vi "Start Regs.vi"(8 "error in (no error)":errorcluster, 9 "Regs_Descriptions":string[][](array[string]), 10 "RegsParam":dbl[][](array[numeric]), 11 "Queue in":T1) -> (0 "error out":errorcluster)   [LabVIEW 2019, in "Reg visu.lvclass"]
uses:
  Reg visu/Reg visu.lvclass
  <vilib>/NI/AMC/Message Queue.ctl
  <vilib>/NI/AMC/Message.ctl
  <vilib>/NI/Tools/Keyed Array/KeyedArray.ctl
  Reg visu/Reg visu.lvclass/Reg visu.ctl
  Reg visu/Run.vi
  <vilib>/NI/Tools/Keyed Array/Tools_KeyedArray.lvlib
  <vilib>/NI/AMC/AMC.lvlib
panel:
  # "group"
  # "process_gas"
  # "fcode"
  # "fcode_full"
  # "instrument_range_max"
  # "auto_value"
  # "alr_value"
  # "output_k"
  # "output_set_time"
  # "process_units"
  # "Names"
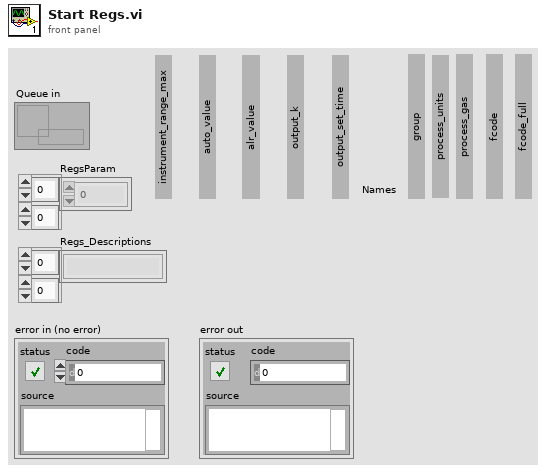
[diagram p1: front panel]
types:
  T1 = typedef "AMC.lvlib/Message Queue.ctl" = refnum<queue>
  T2 = enum32{"Invalid", "Standard", "Closed", "Hidden", "Minimized", "Maximized"}
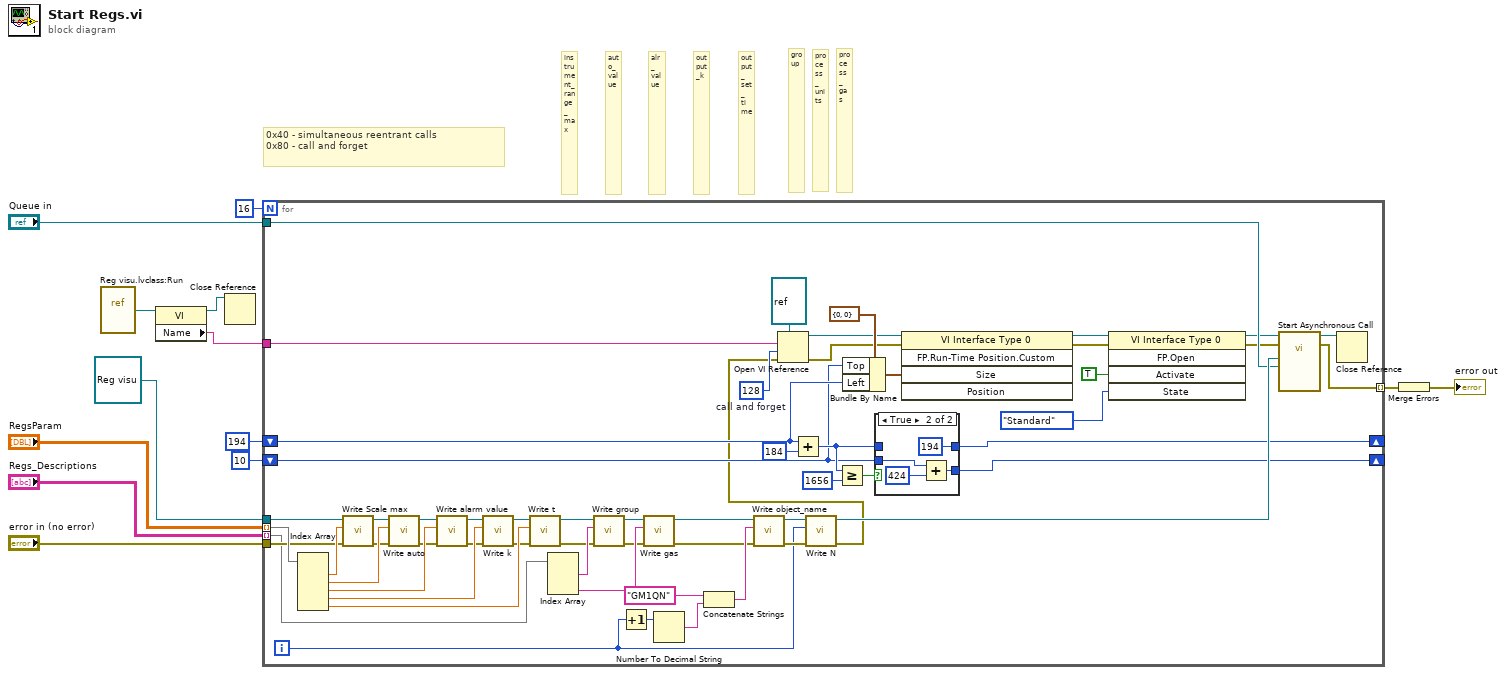
[diagram p0: block diagram]
diagram:
  # "process_gas"
  # "group"
  # "process_units"
  # "output_set_time"
  # "output_k"
  # "alr_value"
  # "instrument_range_max"
  # "auto_value"
  # "0x40 - simultaneous reentrant calls\n0x80 - call and forget"
  n1 = vi-ref "Reg visu.lvclass:Run.vi"() -> (w8:refnum<vi>)
  n2 = property class="VI"(reference=w8) -> (reference out=w7:refnum<vi>, "Name"=w3:string)  [unwired: 1 in, 1 out]
  n3 = Close Reference(reference=w7) -> ()  [unwired: 1 in, 1 out]
  n4 = for {
    N: 16 -> [_]
    tunnel: [w71] -> w9 mode=indexing
    tunnel: refnum<class "Reg visu.lvclass"> refnum ("Reg visu.lvclass") -> [w14]
    tunnel: "Queue in" -> [w63]
    shift-right: [w48] -> _
    shift-left: i16 194 ("x") -> [w50]
    shift-right: [w47] -> _
    shift-left: i16 10 ("x") -> [w49]
    tunnel: "error in (no error)" -> [w32]
    tunnel: w3 -> [w44]
    tunnel: "RegsParam" -> [w34] mode=indexing
    tunnel: "Regs_Descriptions" -> [w23] mode=indexing
    i -> [w64]
    w45 = 128  # call and forget
    n5 = Index Array(array=w34) -> (element #1=w33:dbl, element #2=w31:dbl, element #3=w29:dbl, element #4=w27:dbl, element #5=w25:dbl)  [unwired: 5 in]
    n6 = call "Write Scale max.vi"("error in (no error)"=w32, "Scale max"=w33, "Reg visu in"=w14) -> ("error out"=w30:errorcluster, "Reg visu out"=w38:refnum<class "Reg visu.lvclass">)  [unwired: 7 in]
    n7 = call "Write auto.vi"("error in (no error)"=w30, "auto"=w31, "Reg visu in"=w38) -> ("error out"=w28:errorcluster, "Reg visu out"=w37:refnum<class "Reg visu.lvclass">)  [unwired: 7 in]
    n8 = call "Write alarm value.vi"("error in (no error)"=w28, "alarm value"=w29, "Reg visu in"=w37) -> ("error out"=w26:errorcluster, "Reg visu out"=w36:refnum<class "Reg visu.lvclass">)  [unwired: 7 in]
    n9 = call "Write k.vi"("error in (no error)"=w26, "k"=w27, "Reg visu in"=w36) -> ("error out"=w24:errorcluster, "Reg visu out"=w35:refnum<class "Reg visu.lvclass">)  [unwired: 7 in]
    n10 = call "Write t.vi"("error in (no error)"=w24, "t"=w25, "Reg visu in"=w35) -> ("error out"=w19:errorcluster, "Reg visu out"=w20:refnum<class "Reg visu.lvclass">)  [unwired: 7 in]
    n11 = Index Array(array=w23) -> (element #1=w22:string, element #3=w21:string)  [unwired: 3 in, 1 out]
    n12 = call "Write group.vi"("error in (no error)"=w19, "group"=w22, "Reg visu in"=w20) -> ("error out"=w18:errorcluster, "Reg visu out"=w17:refnum<class "Reg visu.lvclass">)  [unwired: 7 in]
    n13 = Increment(x=w64) -> (x+1=w66:i32)
    n14 = call "Write gas.vi"("error in (no error)"=w18, "gas"=w21, "Reg visu in"=w17) -> ("error out"=w15:errorcluster, "Reg visu out"=w16:refnum<class "Reg visu.lvclass">)  [unwired: 7 in]
    n15 = Number To Decimal String(number=w66) -> (decimal integer string=w65:string)  [unwired: 1 in]
    n16 = Concatenate Strings("GM1QN" ("string"), w65) -> (w42:string)
    n17 = call "Write object_name.vi"("error in (no error)"=w15, "object_name"=w42, "Reg visu in"=w16) -> ("error out"=w68:errorcluster, "Reg visu out"=w69:refnum<class "Reg visu.lvclass">)  [unwired: 7 in]
    n18 = Add(x=w50, y=i16 184) -> (x+y=w56:i16)
    n19 = call "Write N.vi"("error in (no error)"=w68, "N"=w64, "Reg visu in"=w69) -> ("error out"=w39:errorcluster, "Reg visu out"=w70:refnum<class "Reg visu.lvclass">)  [unwired: 7 in]
    n20 = Open VI Reference(type specifier VI Refnum (for type only)=refnum<vi> refnum, vi path=w44, options=w45, error in (no error)=w39) -> (vi reference=w41:refnum<vi>, error out=w40:errorcluster)  [unwired: 2 in]
    n21 = Greater Or Equal?(x=w56, y=i16 1656) -> (x >= y?=w57:bool)
    n22 = Bundle By Name(cluster=cluster{"Top":i16, "Left":i16} {"Top"=0, "Left"=0} ("Position"), "Top"=w49, "Left"=w50) -> (w55:cluster{"Top":i16, "Left":i16})
    n23 = case shown="True" w57 {
      tunnel: w56 -> [w72 _]
      tunnel: [w72 i16 194 ("x")] -> w48
      tunnel: w49 -> [w73 w76]
      tunnel: [w73 w75] -> w47
      frame False {
      }
      frame True {
        n24 = Add(x=w76, y=i16 424) -> (x+y=w75:i16)
      }
    }
    n25 = invoke class="VI Interface Type 0" method="FP.Run-Time Position.Custom"(reference=w41, error in=w40, "Size"=w55) -> (reference out=w54:refnum<vi>, error out=w53:errorcluster)  [unwired: 2 in, 3 out]
    n26 = invoke class="VI Interface Type 0" method="FP.Open"(reference=w54, error in=w53, "Activate"=TRUE ("Activate?"), "State"=T2."Standard") -> (reference out=w52:refnum<vi>, error out=w51:errorcluster)  [unwired: 1 in, 3 out]
    n27 = call-by-ref "Start Asynchronous Call"(reference=w52, error in=w51, "message queue in"=w63, "Reg visu in"=w70) -> (reference out=w43:refnum<vi>, error out=w71:errorcluster)  [unwired: 9 in, 1 out]
    n28 = Close Reference(reference=w43) -> ()  [unwired: 1 in, 1 out]
  }
  n29 = Merge Errors(w9) -> (→"error out":errorcluster)
